vi "ClrFIFO.vi"(11 "FPGA in":refnum<queue>) -> (2 "Table":string[][](array[string]), 3 "FPGA out":refnum<queue>)   [LabVIEW 2019, in "FPGA.lvlib"]
uses:
  FPGA.lvlib
  FPGA.ctl
  Commands.ctl
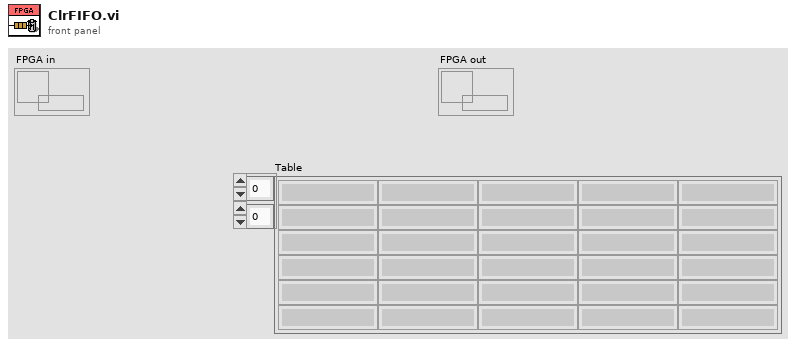
[diagram p1: front panel]
types:
  T1 = typedef "FPGA.lvlib/Commands.ctl" = string
  T2 = cluster{"Start freq. [Hz]":dbl, "Sweep duration [s]":dbl, "Freq. step [Hz]":dbl, "Stop freq. [Hz]":dbl, "Time for step [s]":dbl, "Amplitude [mVpp]":dbl, "Number of steps":i32}[]
  T3 = typedef "FPGA.lvlib/FPGA.ctl" = cluster{"Start freq. [Hz]":dbl, "Sweep duration [s]":dbl, "Freq. step [Hz]":dbl, "DAC Sample Rate":dbl, "ADC Sample Rate":dbl, "CMD port":u16, "DFAST port":u16, "CMD ID":refnum<k16>, "DFAST ID":refnum<k16>, "CMD error out":errorcluster, "FPGA IP":string, "DFAST error out ":errorcluster, "Stop freq. [Hz]":dbl, "Discrete sweep":bool, "Initial NCO":u32, "Difference NCO":i32, "step NCO":i64, "Final NCO":u32, "clocks for step":u32, "demodulation":bool, "NCO Phase Precision":u32, "NCO Sample Rate":dbl, "Time for step [s]":dbl, "NCO freq. resolution":dbl, "Sweep speed [Hz/s]":dbl, "Connected":bool, "Slew Rate [V/us]":dbl, "Parameters_ok":bool, "Amplitude [mVpp]":dbl, "Scale Factor":fxp<+,16,0>, "Acquiring":bool, "DAC-ADC Latency":u16, "Digital Gain":i32, "Number of steps":i32, "Averaging preferred":bool, "Filter Order":u32, "Settling":enum16{"99%", "99,9%"}, "FIFO":cluster{"Start freq. [Hz]":dbl, "Sweep duration [s]":dbl, "Freq. step [Hz]":dbl, "Stop freq. [Hz]":dbl, "Time for step [s]":dbl, "Amplitude [mVpp]":dbl, "Number of steps":i32}[]}
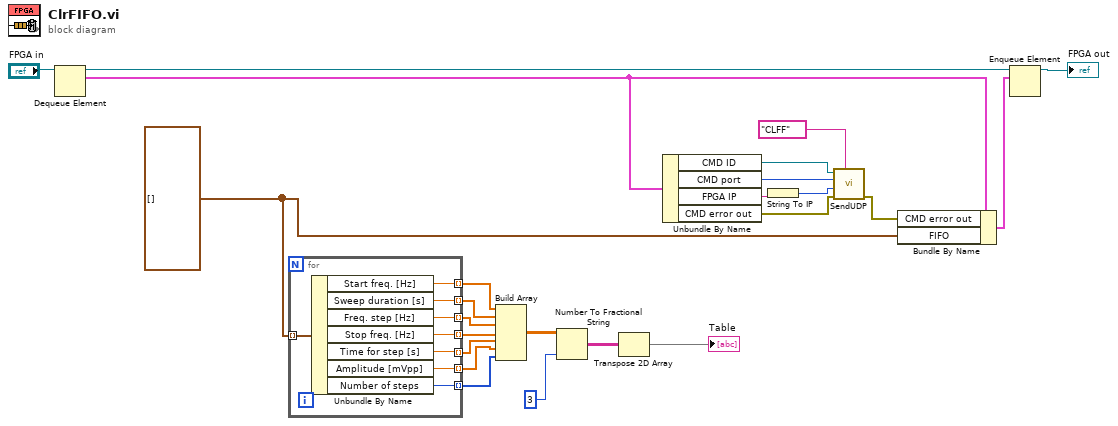
[diagram p0: block diagram]
diagram:
  w9 = T2 [] ("FIFO")
  n1 = Dequeue Element(queue="FPGA in") -> (queue out=w23:refnum<queue>, element=w2:T3)  [unwired: 2 in, 2 out]
  n2 = for {
    tunnel: w9 -> [w32] mode=indexing
    tunnel: [w31] -> w18 mode=indexing
    tunnel: [w30] -> w19 mode=indexing
    tunnel: [w29] -> w20 mode=indexing
    tunnel: [w28] -> w21 mode=indexing
    tunnel: [w27] -> w17 mode=indexing
    tunnel: [w26] -> w16 mode=indexing
    tunnel: [w25] -> w15 mode=indexing
    n3 = Unbundle By Name(w32) -> ("Start freq. [Hz]"=w31:dbl, "Sweep duration [s]"=w30:dbl, "Freq. step [Hz]"=w29:dbl, "Stop freq. [Hz]"=w28:dbl, "Time for step [s]"=w27:dbl, "Amplitude [mVpp]"=w26:dbl, "Number of steps"=w25:i32)
  }
  n4 = Build Array(w18, w19, w20, w21, w17, w16, w15) -> (w14:dbl[][])
  n5 = Number To Fractional String(number=w14, precision (6)=i16 3) -> (F-format string=w12:string[][])  [unwired: 2 in]
  n6 = Transpose 2D Array(2D array=w12) -> (transposed array=→"Table":string[][])
  n7 = Unbundle By Name(w2) -> ("CMD ID"=w6:refnum<k16>, "CMD port"=w5:u16, "FPGA IP"=w7:string, "CMD error out"=w3:errorcluster)
  n8 = String To IP(1:w7) -> (0:w4:u32)
  n9 = call "SendUDP.vi"("data in"=T1 "CLFF" ("Combo Box"), "error in (no error)"=w3, "address"=w4, "port or service name"=w5, "connection ID"=w6) -> ("error out"=w1:errorcluster)  [unwired: 1 in, 5 out]
  n10 = Bundle By Name(cluster=w2, "CMD error out"=w1, "FIFO"=w9) -> (w13:T3)
  n11 = Enqueue Element(queue=w23, element=w13) -> (queue out=→"FPGA out":refnum<queue>)  [unwired: 2 in, 2 out]
